vi "GPS Handler.vi"   [LabVIEW 2020]
uses:
  <vilib>/Platform/TimedLoop/XDataNode/timing_clust.ctl
  <vilib>/Platform/TimedLoop/XDataNode/nitl_modes.ctl
  <vilib>/Platform/TimedLoop/XDataNode/wakeup.ctl
  Type Definitions/Enum - Data.ctl
  Type Definitions/Payload Class.ctl
  Type Definitions/GPS Solution Data.ctl
  <vilib>/Utility/error.llb/Error Cluster From Error Code.vi
  <vilib>/rvi/errors/niLvFpgaAdjustHostInterfaceError.vi
  <vilib>/platform/TimedLoop/XDataNode/XDataNode.xnode
  <vilib>/rvi/interface/nirviReadWriteControl/nirviReadWriteControl.xnode
  <vilib>/Platform/TimedLoop/XDataNode/XDNodeRunTimeDep.lvlib
  NiFpgaLv.dll
  <vilib>/rvi/interface/Simulation/niFpgaSimulationCallBeginRW.vi
types:
  T1 = typedef "System Resources.ctl" = cluster{"System Session":refnum<k21>, "System Resource":refnum<k20>, "FPGA VI Reference":refnum<k20>}
  T2 = typedef "XDNodeRunTimeDep.lvlib/timing_clust.ctl" = cluster{"Expected End [f-1]":u64, "Actual End [f-1]":u64, "Finished Late? [f-1]":bool, "Expected End [i-1]":u64, "Actual End [i-1]":u64, "Finished Late? [i-1]":bool, "Expected Start [i]":u64, "Actual Start [i]":u64, "Expected Start [f]":u64, "Actual Start [f]":u64, "Source Name":string, "Structure Name":string, "Period":i64, "Deadline":i64, "Offset":i64, "Start":i64, "Priority":i32, "Timeout":i32, "Mode":T3, "Wakeup Reason":T4, "Error":errorcluster, "Source Type":string, "Secondary Source Type":string, "Global End Time":u64, "Global Start Time":u64, "Frame Duration":u64, "Iteration Duration":u64, "Assigned CPU":i32, "I/O Scan Engine Mode":u32}
  T3 = typedef "XDNodeRunTimeDep.lvlib/nitl_modes.ctl" = enum32{"No Change", "Process missed periods, maintain original phase", "Discard missed periods, maintain original phase", "Process missed periods, ignore original phase", "Discard missed periods, ignore original phase"}
  T4 = typedef "XDNodeRunTimeDep.lvlib/wakeup.ctl" = enum32{"Normal", "Aborted", "Asynchronous wakeup", "Timing source error", "Timed loop error", "Timeout"}
  T5 = typedef "GPS Solution Data.ctl" = cluster{"GPS Timestamp":timestamp, "GPS Status":enum8{"Initializing", "Normal", "Unable to get fix"}, "GPS Antenna Status":enum8{"Unknown", "Normal", "Absent", "Overcurrent"}, "GPS Satelites Available":u8, "GPS Time Lock":bool, "GPS UTC Offset Valid":bool, "GPS Self-Survey Complete":bool, "GPS Latitude (°)":dbl, "GPS Longitude (°)":dbl, "GPS Altitude (m)":dbl, "GPS Serial Number":u32, "GPS Vendor ID":u16, "GPS Firmware Version":u32}
  T6 = typedef "Payload Class.ctl" = enum16{"System State", "Parameters", "Metadata", "Software Monitor", "Data", "Commands"}
  T7 = typedef "Enum - Data.ctl" = enum16{"Analog Input Data", "Notification Data", "Analog Output Data", "Digital Output Data", "Command Ack", "Digital Input Data", "GPS Solution Data"}
  T8 = enum8{"Initializing", "Normal", "Unable to get fix"}
  T9 = enum8{"Unknown", "Normal", "Absent", "Overcurrent"}
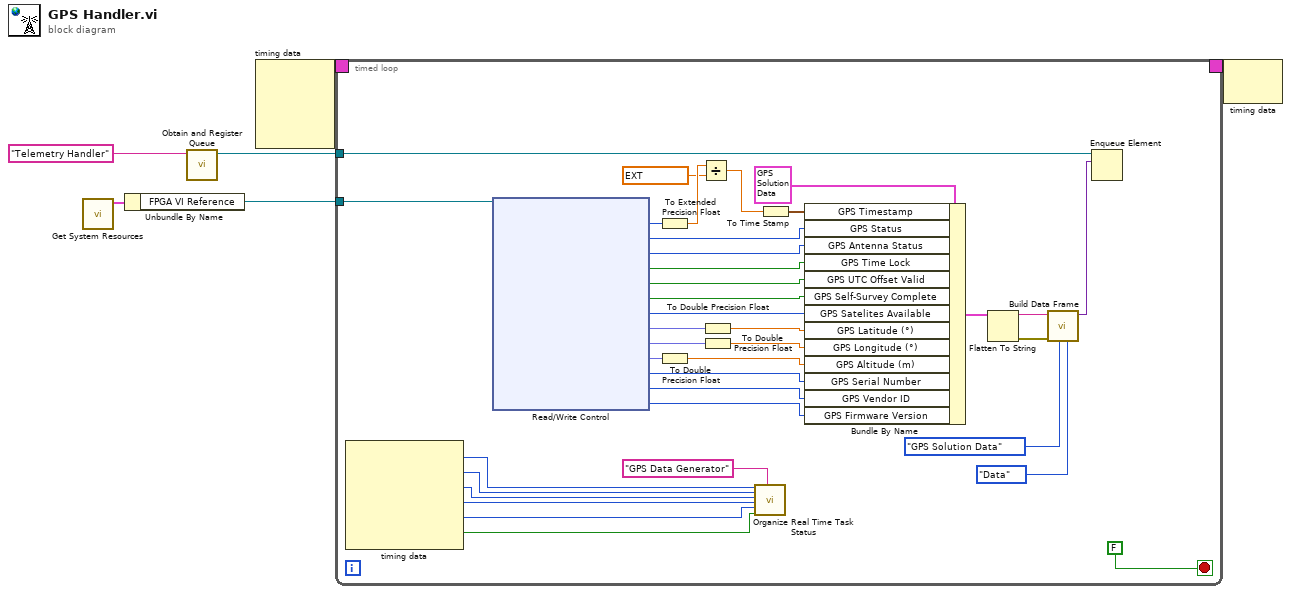
[diagram p0: block diagram]
diagram:
  n1 = call "Get System Resources.vi"() -> ("System Resources"=w2:T1)  [unwired: 10 in, 1 out]
  n2 = Unbundle By Name(w2) -> ("FPGA VI Reference"=w1:refnum<k20>)
  n3 = call "Obtain and Register Queue.vi"("name (unnamed)"="Telemetry Handler") -> ("Queue Out"=w3:refnum<queue>)  [unwired: 7 in, 3 out]
  n4 = node-c288() -> (w6:T2)  [unwired: 4 in]
  n5 = timed-loop {
    timing: w6 -> [_]
    timing-out: [_] -> w5
    tunnel: w3 -> [w29]
    tunnel: w1 -> [w35]
    stop <- FALSE stop-if-true
    n6 = node-c288() -> (w41:i32, w40:i32, w39:i64, w38:i64, w37:i64, w36:bool)  [unwired: 1 in]
    n7 = xnode "Read/Write Control"("FPGA VI Reference In"=w35) -> ("GPS Time (ns)"=w28:u64, "GPS Status"=w19:T8, "GPS Antenna Status"=w18:T9, "GPS Time Lock"=w17:bool, "GPS UTC Offset Valid"=w16:bool, "GPS Self-Survey Complete"=w15:bool, "GPS Satelites Available"=w7:u8, "GPS Latitude (°)"=w24:fxp<+/-,28,8>, "GPS Longitude (°)"=w23:fxp<+/-,29,9>, "GPS Altitude (m)"=w22:fxp<+/-,24,17>, "GPS Serial Number"=w12:u32, "GPS Vendor ID"=w11:u16, "GPS Firmware Version"=w10:u32)  [unwired: 1 in, 2 out]
    n8 = To Extended Precision Float(1:w28) -> (0:w27:ext)
    n9 = To Double Precision Float(number=w22) -> (double precision float=w13:dbl)
    n10 = Divide(x=w27, y=ext 1000000000.0) -> (x/y=w25:ext)
    n11 = To Double Precision Float(number=w24) -> (double precision float=w8:dbl)
    n12 = To Double Precision Float(number=w23) -> (double precision float=w14:dbl)
    n13 = call "Organize Real Time Task Status.vi"("Priority"=w41, "Processor"=w40, "Offset"=w39, "Iteration Duration"=w38, "Period"=w37, "Finished Late? [i-1]"=w36, "Task Name"="GPS Data Generator") -> ()  [unwired: 12 in, 1 out]
    n14 = To Time Stamp(1:w25) -> (0:w20:timestamp)
    n15 = Bundle By Name(cluster=T5 {"GPS Timestamp"=timestamp(0 s since 1904-01-01), "GPS Status"=enum."Initializing", "GPS Antenna Status"=enum."Unknown", "GPS Satelites Available"=0, "GPS Time Lock"=FALSE, "GPS UTC Offset Valid"=FALSE, "GPS Self-Survey Complete"=FALSE, "GPS Latitude (°)"=0.0, "GPS Longitude (°)"=0.0, "GPS Altitude (m)"=0.0, "GPS Serial Number"=0, "GPS Vendor ID"=0, "GPS Firmware Version"=0} ("Cluster"), "GPS Timestamp"=w20, "GPS Status"=w19, "GPS Antenna Status"=w18, "GPS Time Lock"=w17, "GPS UTC Offset Valid"=w16, "GPS Self-Survey Complete"=w15, "GPS Satelites Available"=w7, "GPS Latitude (°)"=w8, "GPS Longitude (°)"=w14, "GPS Altitude (m)"=w13, "GPS Serial Number"=w12, "GPS Vendor ID"=w11, "GPS Firmware Version"=w10) -> (w9:T5)
    n16 = Flatten To String(anything=w9) -> (data string=w31:string, error out=w33:errorcluster)  [unwired: 3 in, 1 out]
    n17 = call "Build Data Frame.vi"("Payload Class (Data)"=Payload_Class."Data", "Payload ID (0)"=Enum_-_Data."GPS Solution Data" ("Data"), "error in (no error)"=w33, "Payload (Empty String)"=w31) -> ("Frame"=w30:variant)  [unwired: 6 in, 1 out]
    n18 = Enqueue Element(queue=w29, element=w30) -> ()  [unwired: 2 in, 3 out]
  }
  n19 = node-c288(w5) -> ()  [unwired: 1 out]
